vi "Video_FlipFrameBuffer.vi"() -> (3 "New Offscreen Buffer":u8)   [LabVIEW 2020]
uses:
  <vilib>/Platform/TimedLoop/XDataNode/timing_clust.ctl
  <vilib>/Platform/TimedLoop/XDataNode/nitl_modes.ctl
  <vilib>/Platform/TimedLoop/XDataNode/wakeup.ctl
  <vilib>/Utility/error.llb/Clear Errors.vi
  <vilib>/rvi/Emulation/niFpgaSctlEmulationGetInTimedLoop.vi
  <vilib>/rvi/Emulation/niFpgaEmulationIsFPGAContextNoSignature.vi
  <vilib>/rvi/DataTransferAndStorage/Container/Common/niFpgaContainerGetUniqueNameForEmu.vi
  <vilib>/rvi/Memory/Memory_Emulation/niFpgaMemoryEmulationCacheClearOnFirstRun.vi
  <vilib>/rvi/Memory/Memory_Emulation/nirvimemoryEmulationManagerCache_MakeExclusive.vi
  <vilib>/rvi/Memory/Memory_Emulation/niFpgaMemoryEmulationValidateCache.vi
  <vilib>/rvi/Memory/Memory_Emulation/nirvimemoryEmulationManagerCache_InsertValue.vi
  <vilib>/rvi/Memory/Memory_Emulation/nirvimemoryEmulationManagerCache_ReleaseExclusive.vi
  <vilib>/rvi/Memory/Memory_Emulation/nirvimemoryEmulationManagerCache_GetValue.vi
  <vilib>/rvi/Memory/Memory_Emulation/nirvimemoryEmulationManagerCache_SetValue.vi
  <vilib>/rvi/Emulation/niFpgaProcessEmulError.vi
  <vilib>/rvi/DataTransferAndStorage/Container/XNode/niFpgaContainer.xnode
  <vilib>/rvi/DataTransferAndStorage/Register/Emulation/niFpgaRegisterEmulation.vi
  <vilib>/Platform/TimedLoop/XDataNode/XDataNode.xnode
  <vilib>/Platform/TimedLoop/XDataNode/XDNodeRunTimeDep.lvlib
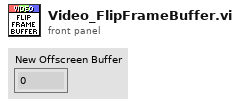
[diagram p1: front panel]
types:
  T1 = typedef "XDNodeRunTimeDep.lvlib/timing_clust.ctl" = cluster{"Expected End [f-1]":u64, "Actual End [f-1]":u64, "Finished Late? [f-1]":bool, "Expected End [i-1]":u64, "Actual End [i-1]":u64, "Finished Late? [i-1]":bool, "Expected Start [i]":u64, "Actual Start [i]":u64, "Expected Start [f]":u64, "Actual Start [f]":u64, "Source Name":string, "Structure Name":string, "Period":i64, "Deadline":i64, "Offset":i64, "Start":i64, "Priority":i32, "Timeout":i32, "Mode":T2, "Wakeup Reason":T3, "Error":errorcluster, "Source Type":string, "Secondary Source Type":string, "Global End Time":u64, "Global Start Time":u64, "Frame Duration":u64, "Iteration Duration":u64, "Assigned CPU":i32, "I/O Scan Engine Mode":u32}
  T2 = typedef "XDNodeRunTimeDep.lvlib/nitl_modes.ctl" = enum32{"No Change", "Process missed periods, maintain original phase", "Discard missed periods, maintain original phase", "Process missed periods, ignore original phase", "Discard missed periods, ignore original phase"}
  T3 = typedef "XDNodeRunTimeDep.lvlib/wakeup.ctl" = enum32{"Normal", "Aborted", "Asynchronous wakeup", "Timing source error", "Timed loop error", "Timeout"}
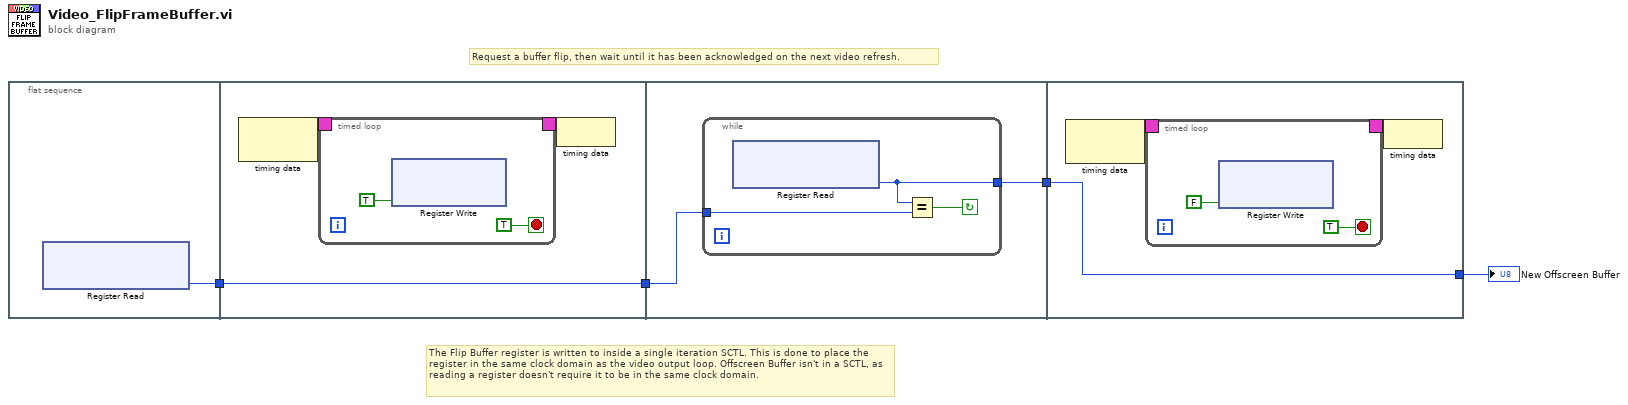
[diagram p0: block diagram]
diagram:
  # "The Flip Buffer register is written to inside a single iteration SCTL. This is done to place the register in the same clock domain as the video output loop. Offscreen Buffer isn't in a SCTL, as reading a register doesn't require it to be in the same clock domain."
  # "Request a buffer flip, then wait until it has been acknowledged on the next video refresh."
  n1 = flat-sequence {
    tunnel: [w5] -> w3
    tunnel: [w6] -> w4
    tunnel: w3 -> [w6]
    tunnel: w4 -> [w16]
    tunnel: [w15] -> w2
    tunnel: w2 -> [w20]
    tunnel: [w20] -> w1
    frame #0 {
      n2 = xnode ("Register Read")() -> ("Data"=w5:u8)  [unwired: 1 in, 1 out]
    }
    frame #1 {
      n3 = node-c288() -> (w8:T1)  [unwired: 1 in]
      n4 = timed-loop {
        timing: w8 -> [_]
        timing-out: [_] -> w7
        stop <- TRUE stop-if-true
        n5 = xnode "Register Write"("Data"=TRUE) -> ()  [unwired: 1 in, 1 out]
      }
      n6 = node-c288(w7) -> ()
    }
    frame #2 {
      n7 = while {
        tunnel: w16 -> [w19]
        tunnel: [w17] -> w15
        stop <- w18 continue-if-true
        n8 = xnode ("Register Read")() -> ("Data"=w17:u8)  [unwired: 1 in, 1 out]
        n9 = Equal?(x=w17, y=w19) -> (x = y?=w18:bool)
      }
    }
    frame #3 {
      n10 = node-c288() -> (w22:T1)  [unwired: 1 in]
      n11 = timed-loop {
        timing: w22 -> [_]
        timing-out: [_] -> w21
        stop <- TRUE stop-if-true
        n12 = xnode "Register Write"("Data"=FALSE) -> ()  [unwired: 1 in, 1 out]
      }
      n13 = node-c288(w21) -> ()
    }
  }
  "New Offscreen Buffer" <- w1
